vi "QPSK.vi"() -> ()   [LabVIEW 2012]
uses:
  <vilib>/express/express analysis/Spectral/Block/exnSpectralBlock spectral measurements PSD poly.vi
  <vilib>/express/express analysis/Spectral/Block/exnSpectralBlock spectral measurements PSD WFM.vi
  <vilib>/express/express analysis/Spectral/XNode/ExpressSpectralMeasurementsBlockNode.xnode
  <vilib>/Analysis/NI_AALPro.lvlib
panel:
  out "Waveform Graph":cluster{"f0":dbl, "df":dbl, "magnitude":dbl[]}(graph)
  out "qpsk":dbl[](graph)
  out "Waveform Chart 2":dbl(graph)
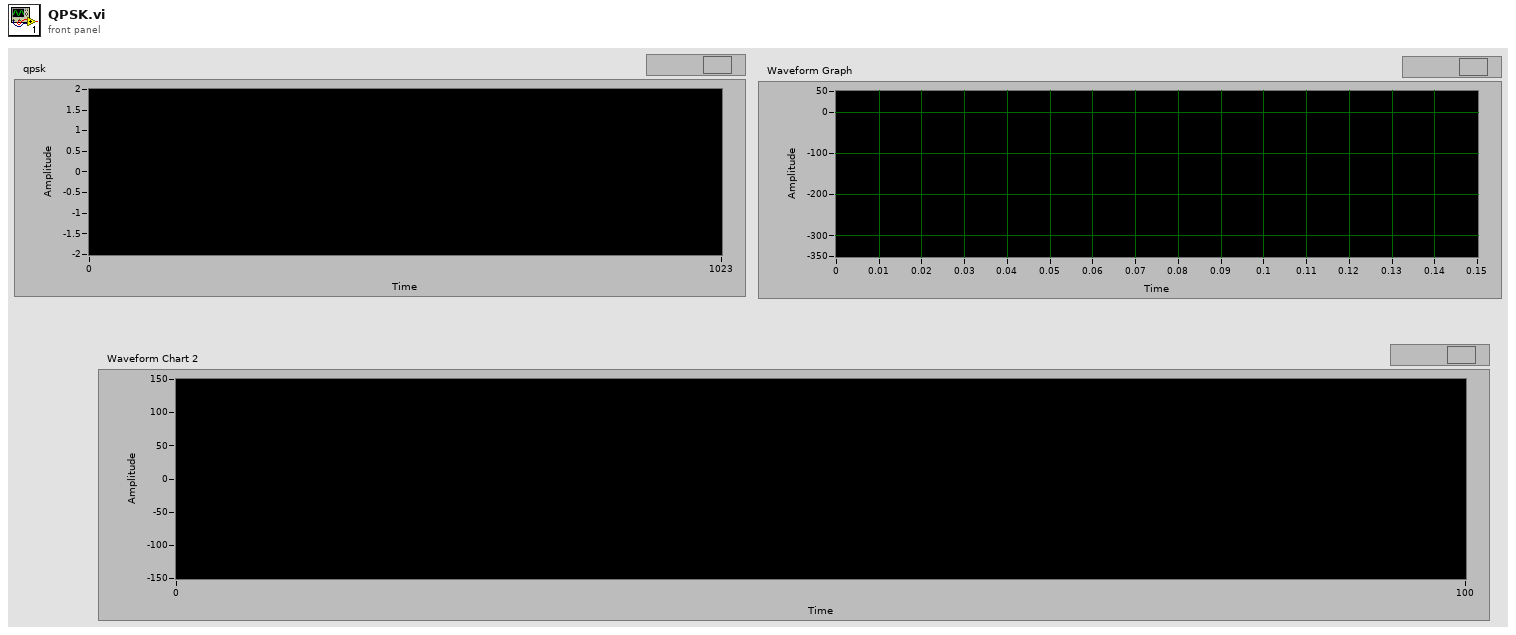
[diagram p1: front panel]
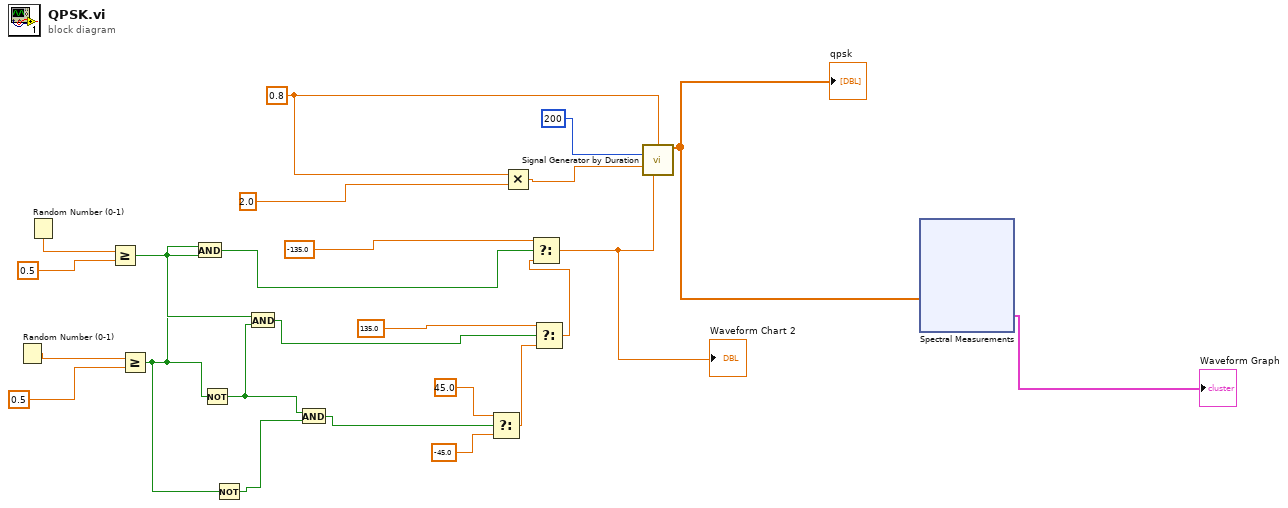
[diagram p0: block diagram]
diagram:
  w5 = 0.8 ("x")
  n1 = Random Number (0-1)() -> (number: 0 to 1=w18:dbl)
  n2 = Random Number (0-1)() -> (number: 0 to 1=w20:dbl)
  n3 = Greater Or Equal?(x=w20, y=0.5) -> (x >= y?=w15:bool)
  n4 = Greater Or Equal?(x=w18, y=0.5) -> (x >= y?=w13:bool)
  n5 = And(x=w13, y=w15) -> (x .and. y?=w16:bool)
  n6 = Not(x=w13) -> (.not. x?=w8:bool)
  n7 = Not(x=w13) -> (.not. x?=w7:bool)
  n8 = And(x=w15, y=w8) -> (x .and. y?=w14:bool)
  n9 = And(x=w8, y=w7) -> (x .and. y?=w9:bool)
  n10 = Select(t=45.0, s=w9, f=-45.0) -> (s? t:f=w12:dbl)
  n11 = Multiply(x=w5, y=2.0) -> (x*y=w2:dbl)
  n12 = Select(t=135.0, s=w14, f=w12) -> (s? t:f=w22:dbl)
  n13 = Select(t=-135.0, s=w16, f=w22) -> (s? t:f=w4:dbl)
  "Waveform Chart 2" <- w4
  n14 = call <vilib>:"Signal Generator by Duration.vi"("duration"=w5, "# of samples"=200, "amplitude"=w2, "phase in"=w4) -> ("signal"=w3:dbl[])  [unwired: 8 in, 3 out]
  "qpsk" <- w3
  n15 = xnode "Spectral Measurements"("Signals"=w3) -> ("PSD"=→"Waveform Graph":cluster{"f0":dbl, "df":dbl, "magnitude":dbl[]})  [unwired: 1 in, 1 out]
